vi "Calc Text Size.vi"(11 "State In":T1) -> (3 "State":T1)   [LabVIEW 2020, in "FlexBlock.xnode"]
uses:
  FlexBlock.xnode
  State.ctl
  FlexBlocks/Type Descriptor.ctl
  FlexBlocks/Terminal Direction.ctl
  FlexBlocks/Value Mode.ctl
  FlexBlocks/Terminal State.ctl
  FlexBlocks/Special Terminal.ctl
  FlexBlocks/Errors.ctl
  <vilib>/picture/picture.llb/imagedata.ctl
  FlexBlocks/Calculated Sizes.ctl
  FlexBlocks/FlexBlocks.lvlib
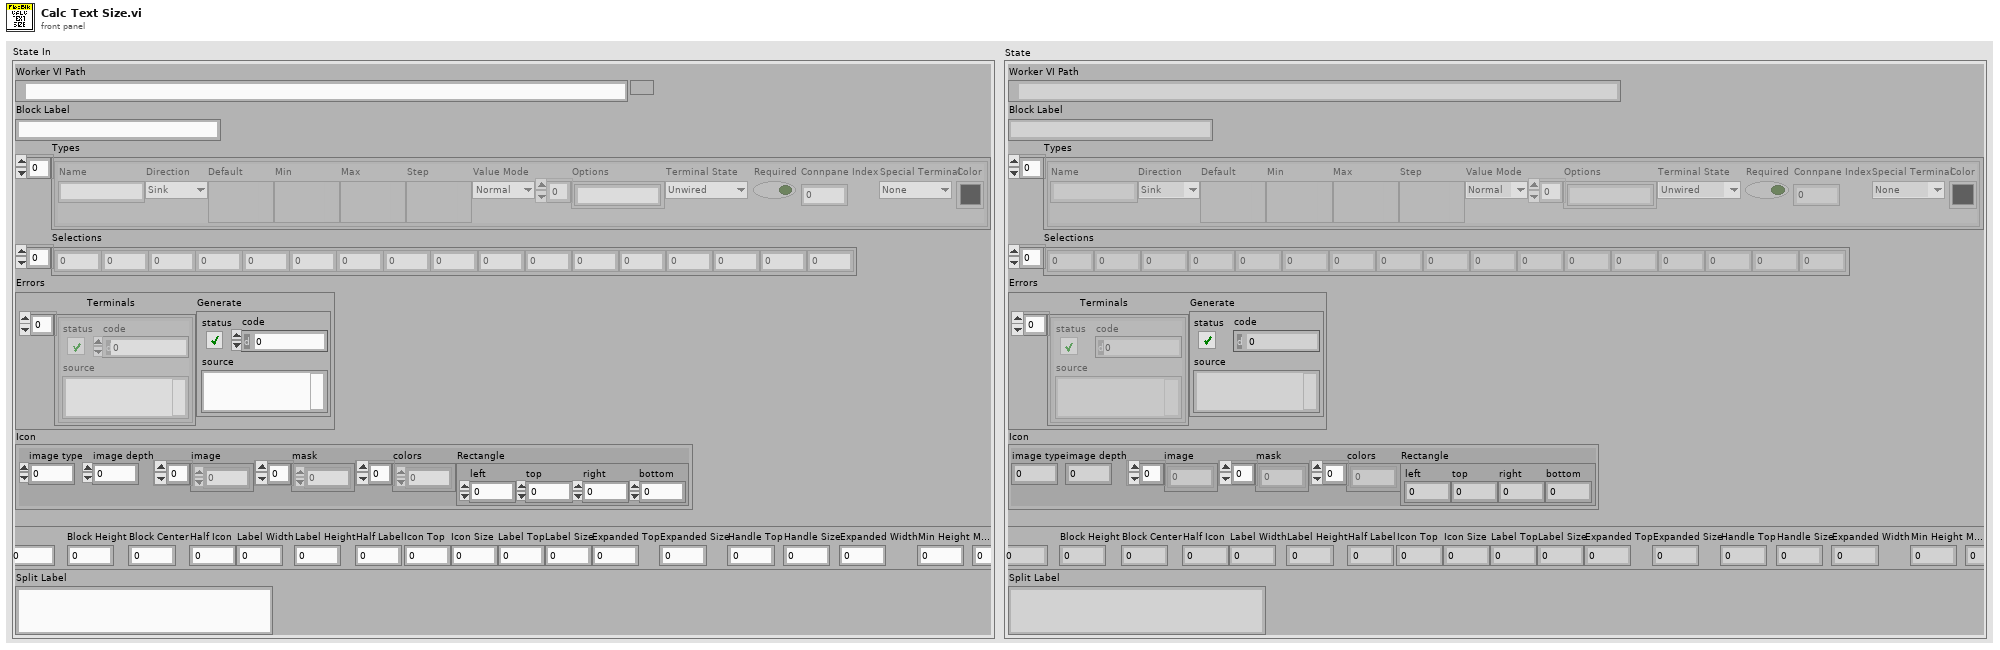
[diagram p1: front panel]
types:
  T1 = typedef "FlexBlock.xnode/State.ctl" = cluster{"Worker VI Path":path, "Block Label":string, "Types":T2[], "Selections":i32[], "Errors":T7, "Icon":T8, "Calcd Sizes":T9, "Split Label":string}
  T2 = typedef "FlexBlocks.lvlib/Type Descriptor.ctl" = cluster{"Name":string, "Direction":T3, "Default":variant, "Min":variant, "Max":variant, "Step":variant, "Value Mode":T4, "Options":string[], "Terminal State":T5, "Required":bool, "Connpane Index":i32, "Special Terminal":T6, "Color":u32}
  T3 = typedef "FlexBlocks.lvlib/Terminal Direction.ctl" = enum16{"Sink", "Source"}
  T4 = typedef "FlexBlocks.lvlib/Value Mode.ctl" = enum16{"Normal", "Range", "Select"}
  T5 = typedef "FlexBlocks.lvlib/Terminal State.ctl" = enum16{"Unwired", "BadType", "BadRef", "Channel", "Value", "Control Ref"}
  T6 = typedef "FlexBlocks.lvlib/Special Terminal.ctl" = enum16{"None", "Action", "Init", "Tag", "State in", "State out", "Error"}
  T7 = typedef "FlexBlocks.lvlib/Errors.ctl" = cluster{"Terminals":errorcluster[], "Generate":errorcluster}
  T8 = typedef "imagedata.ctl" = cluster{"image type":i32, "image depth":i32, "image":u8[], "mask":u8[], "colors":u32[], "Rectangle":cluster{"left":i16, "top":i16, "right":i16, "bottom":i16}}
  T9 = typedef "FlexBlocks.lvlib/Calculated Sizes.ctl" = cluster{"Text Width":i32, "Text Height":i32, "Half Text":i32, "Block Width":i32, "Block Height":i32, "Block Center":i32, "Half Icon":i32, "Label Width":i32, "Label Height":i32, "Half Label":i32, "Icon Top":i32, "Icon Size":i32, "Label Top":i32, "Label Size":i32, "Expanded Top":i32, "Expanded Size":i32, "Handle Top":i32, "Handle Size":i32, "Expanded Width":i32, "Min Height":i32, "Max Height":i32}
  T10 = typedef "FlexBlocks.lvlib/Size Constants.ctl" = cluster{"Icon":i32, "Value Width":i32, "BG Rounding":i32, "Term Width":i32, "Term Height":i32, "Text Offset":i32, "Value Padding":i32, "Select Padding":i32, "Min Block Width":i32, "Vertical Margin":i32, "Size Handle Height":i32, "Name Padding":i32}
  T11 = cluster{"left":i16, "top":i16, "right":i16, "bottom":i16}
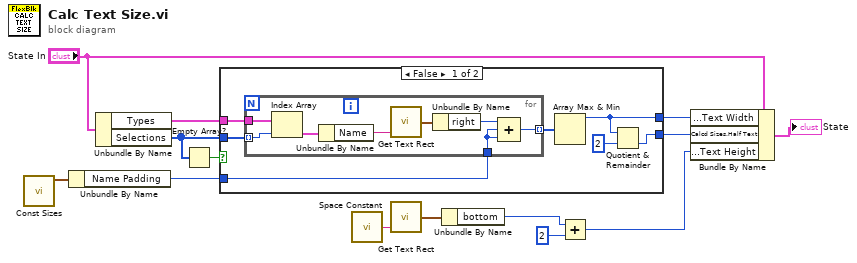
[diagram p0: block diagram]
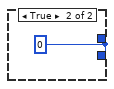
[diagram p2: hidden frame]
diagram:
  n1 = call "Const Sizes.vi"() -> ("Sizes"=w2:T10)  [unwired: 11 in]
  n2 = Unbundle By Name(w2) -> ("Name Padding"=w1:i32)
  n3 = Unbundle By Name("State In") -> ("Types"=w14:T2[], "Selections"=w9:i32[])
  n4 = Empty Array?(array=w9) -> (empty?=w8:bool)
  n5 = case shown="False" w8 {
    tunnel: w14 -> [w21 _]
    tunnel: [w19 w30] -> w12
    tunnel: [w17 w30] -> w11
    tunnel: w9 -> [w16 _]
    tunnel: w1 -> [w15 _]
    frame False {
      n6 = for {
        tunnel: w21 -> [w29]
        tunnel: [w23] -> w20 mode=indexing
        tunnel: w16 -> [w24] mode=indexing
        tunnel: w15 -> [w22]
        n7 = Index Array(array=w29, index=w24) -> (element=w25:T2)
        n8 = Unbundle By Name(w25) -> ("Name"=w28:string)
        n9 = call <vilib>:"Get Text Rect.vi"("text"=w28) -> ("rect"=w27:T11)  [unwired: 8 in]
        n10 = Unbundle By Name(w27) -> ("right"=w26:i16)
        n11 = Compound Arithmetic op=unknown(w26, w22, w22) -> (w23:i32)
      }
      n12 = Array Max & Min(array=w20) -> (max value=w19:i32)  [unwired: 3 out]
      n13 = Quotient & Remainder(x=w19, y=i16 2) -> (floor(x/y)=w17:i32)  [unwired: 1 out]
    }
    frame True {
      w30 = i16 0
    }
  }
  n14 = call <vilib>:"Space Constant.vi"() -> ("String"=w7:string)
  n15 = call <vilib>:"Get Text Rect.vi"("text"=w7) -> ("rect"=w6:T11)  [unwired: 8 in]
  n16 = Unbundle By Name(w6) -> ("bottom"=w5:i16)
  n17 = Add(x=w5, y=i16 2) -> (x+y=w3:i16)
  n18 = Bundle By Name(cluster="State In", "Calcd Sizes.Text Width"=w12, "Calcd Sizes.Half Text"=w11, "Calcd Sizes.Text Height"=w3) -> (→"State":T1)
